vi "Set Network Settings.vi"(8 "error in":errorcluster, 10 "Network Settings":T1={"IP adress"="0.0.0.0", "RDB"={"Protocol"=enum."UDP", "Tx Port"=48191, "Rx Port"=48190, "Buffer Size"=204800, "Timeout"=10}, "SCP"={"Protocol"=enum."TCP", "Tx Port"=48179, "Rx Port"=48179, "Buffer Size"=204800, "Timeout"=60}}, 11 "Item Ref in":T3 format="%.0x") -> (0 "error out":errorcluster, 3 "Item Ref out":T3 format="%.0x")   [LabVIEW 2023, in "Vires VTD System Explorer.lvlib"]
uses:
  Vires VTD System Explorer.lvlib
  <vilib>/NI VeriStand/Custom Device API/Custom Device Item Ref.ctl
  Shared/Network Settings.ctl
  Shared/Protocol.ctl
  <vilib>/NI VeriStand/Custom Device Tools/Custom Device Utility Library/Search Direction.ctl
  Shared/Constants.vi
  <vilib>/NI VeriStand/Custom Device Tools/Custom Device Utility Library/NI VeriStand - Search for Item by GUID.vi
  <vilib>/NI VeriStand/Custom Device API/Set Item Property (Variant).vi
  Shared/Vires VTD Shared.lvlib
  <vilib>/NI VeriStand/Custom Device API/Custom Device API.lvlib
  <vilib>/NI VeriStand/Custom Device Tools/Custom Device Utility Library/Custom Device Utility Library.lvlib
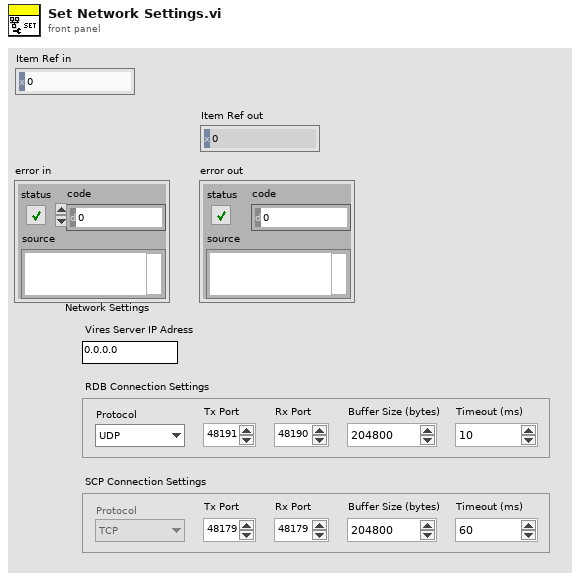
[diagram p1: front panel]
types:
  T1 = typedef "Vires VTD Shared.lvlib/Network Settings.ctl" = cluster{"IP adress":string, "RDB":cluster{"Protocol":T2, "Tx Port":u16, "Rx Port":u16, "Buffer Size":i32, "Timeout":u16}, "SCP":cluster{"Protocol":T2, "Tx Port":u16, "Rx Port":u16, "Buffer Size":i32, "Timeout":u16}}
  T2 = typedef "Vires VTD Shared.lvlib/Protocol.ctl" = enum16{"UDP", "TCP"}
  T3 = typedef "Custom Device API.lvlib/Custom Device Item Ref.ctl" = u64
  T4 = typedef "Custom Device API.lvlib/Custom Device Item Info.ctl" = cluster{"Name":string, "Is Channel":bool, "GUID":string, "Is Waveform":bool}
  T5 = typedef "Custom Device Utility Library.lvlib/Search Direction.ctl" = enum16{"Down", "Up"}
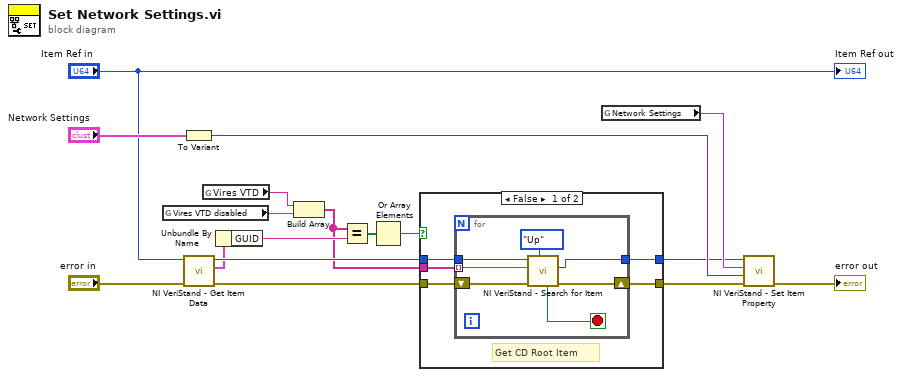
[diagram p0: block diagram]
diagram:
  n1 = global read "Constants.vi" "Vires VTD disabled"() -> (w10:string)
  n2 = To Variant(anything="Network Settings") -> (Variant=w16:variant)
  n3 = call <vilib>:"NI VeriStand - Get Item Data.vi"("error in (no error)"="error in", "Item Ref in"="Item Ref in") -> ("error out"=w13:errorcluster, "Item Info"=w11:T4, "Item Ref out"=w12:T3)  [unwired: 6 in, 1 out]
  n4 = global read "Constants.vi" "Vires VTD"() -> (w9:string)
  n5 = Unbundle By Name(w11) -> ("GUID"=w8:string)
  n6 = Build Array(w9, w10) -> (w5:string[])
  n7 = Equal?(x=w5, y=w8) -> (x = y?=w7:bool[])
  n8 = Or Array Elements(Boolean array=w7) -> (logical OR=w6:bool)
  n9 = case shown="False" w6 {
    tunnel: w13 -> [w22 w31]
    tunnel: [w21 w31] -> w2
    tunnel: [w20 w30] -> w3
    tunnel: w12 -> [w19 w30]
    tunnel: w5 -> [w18 _]
    frame False {
      # "Get CD Root Item"
      n10 = for {
        shift-right: [w27] -> w21
        shift-left: w22 -> [w28]
        tunnel: w18 -> [w24] mode=indexing
        tunnel: w19 -> [w25]
        tunnel: [w26] -> w20
        stop <- w23 stop-if-true
        n11 = call-poly <vilib>:"NI VeriStand - Search for Item.vi"("Direction (Down)"=Search_Direction."Up", "error in"=w28, "Item GUID"=w24, "Section Ref in"=w25) -> ("error out"=w27:errorcluster, "Item Ref"=w26:T3, "Found"=w23:bool)  [unwired: 4 in, 1 out]
      }
    }
    frame True {
      # "Item Ref in is CD Root Item"
    }
  }
  n12 = global read "Constants.vi" "Network Settings"() -> (w17:string)
  n13 = call-poly <vilib>:"NI VeriStand - Set Item Property.vi"("error in (no error)"=w2, "Value"=w16, "Property Name"=w17, "Item Ref in"=w3) -> ("error out"=→"error out":errorcluster)  [unwired: 5 in, 2 out]
  "Item Ref out" <- "Item Ref in"
